vi "LogAndClearError.vi"(7 "Log and view ?":T2, 8 "error in (no error)":errorcluster, 9 "type of dialog":T1 items=["no dialog", "OK message", "continue or stop message", "OK message + warnings", "continue/stop + warnings"]) -> (0 "error out":errorcluster)   [LabVIEW 2011]
uses:
  Ctrls/enumLogAndView.ctl
  <vilib>/Utility/error.llb/DialogType.ctl
  030 - EVENTS/03 - ToMessageHandlerProcess/enumMessageCriticity.ctl
  030 - EVENTS/03 - ToMessageHandlerProcess/ToMessageHandlerEvent.ctl
  030 - EVENTS/EnumFgvEventCommand.ctl
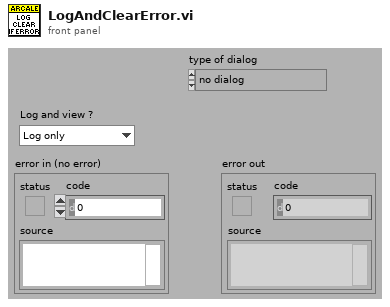
[diagram p1: front panel]
types:
  T1 = typedef "DialogType.ctl" = u16
  T2 = typedef "enumLogAndView.ctl" = enum16{"Log only", "Log and view"}
  T3 = typedef "enumMessageCriticity.ctl" = enum16{"No error", "Info", "Warning", "Error", "Fatal error"}
  T4 = typedef "ToMessageHandlerEvent.ctl" = cluster{"date / time":timestamp, "Criticity":T3, "Emitter":string, "Message":string}
  T5 = typedef "EnumFgvEventCommand.ctl" = enum16{"Setup", "Cleanup", "Get"}
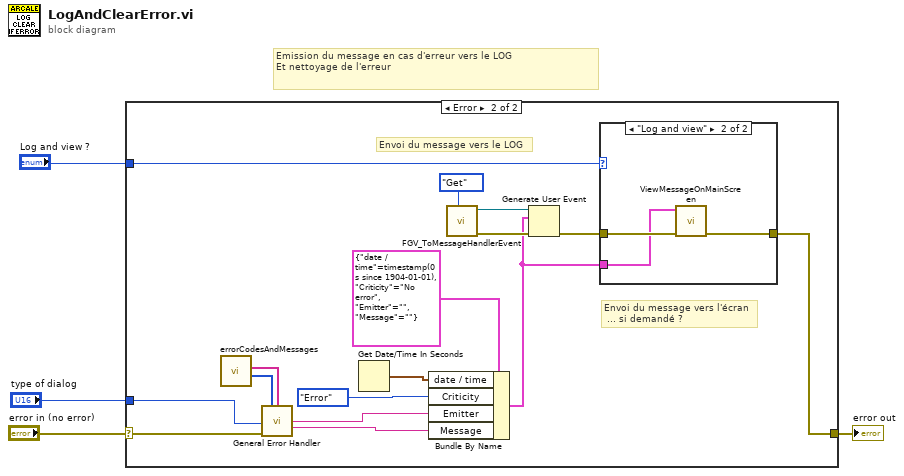
[diagram p0: block diagram]
diagram:
  # "Emission du message en cas d'erreur vers le LOG\nEt nettoyage de l'erreur"
  n1 = case shown="Error" "error in (no error)" {
    selector: "error in (no error)" -> [w5 w18]
    tunnel: [w5 w8] -> w3
    tunnel: "Log and view ?" -> [_ w10]
    tunnel: "type of dialog" -> [_ w6]
    frame No Error {
    }
    frame Error {
      # "Envoi du message vers l'écran\n ... si demandé ?"
      # "Envoi du message vers le LOG"
      n2 = call "errorCodesAndMessages.vi"() -> ("errorCodes"=w20:i32[], "errorMessages"=w19:string[])  [unwired: 10 out]
      n3 = call <vilib>:"General Error Handler.vi"("[user-defined codes]"=w20, "[user-defined descriptions]"=w19, "type of dialog (OK msg:1)"=w6, "error in (no error)"=w18) -> ("source out"=w12:string, "message"=w11:string)  [unwired: 10 out]
      n4 = Get Date/Time In Seconds() -> (seconds since 1Jan1904=w14:timestamp)
      n5 = Bundle By Name(cluster=T4 {"date / time"=timestamp(0 s since 1904-01-01), "Criticity"=enum."No error", "Emitter"="", "Message"=""} ("event data"), "date / time"=w14, "Criticity"=enumMessageCriticity."Error", "Emitter"=w12, "Message"=w11) -> (w7:T4)
      n6 = call "FGV_ToMessageHandlerEvent.vi"("Command"=EnumFgvEventCommand."Get") -> ("error out"=w17:errorcluster, "To message handler event"=w16:refnum<user-event>)  [unwired: 9 in]
      n7 = Generate User Event(user event=w16, event data cluster=w7, error in=w17) -> (error out=w9:errorcluster)  [unwired: 1 out]
      n8 = case shown="\"Log and view\"" w10 {
        tunnel: w9 -> [w22 w25]
        tunnel: [w22 w24] -> w8
        tunnel: w7 -> [_ w23]
        frame "Log only" {
        }
        frame "Log and view" {
          n9 = call "ViewMessageOnMainScreen.vi"("error in (no error)"=w25, "Message"=w23) -> ("error out"=w24:errorcluster)  [unwired: 9 in]
        }
      }
    }
  }
  "error out" <- w3
